vi "HELP.vi"(0 "System no.":i32=1 min=1 max=4 step=1, 5 "error in":errorcluster) -> (14 "Help string":string, 19 "error out":errorcluster)   [LabVIEW 2026]
doc: "Returns help string.\n\nF-206, M-8X0: Only for GCS syntax version = GCS 1.0 (Check with CSV?.vi. If CSV?.vi is not supported, syntax version is GCS 1.0). For GCS 2.0 use HLP?.vi instead."
uses:
  GeneralCommands/Controller names.ctl
  Communication/Syntax.ctl
  Communication/Global1.vi
  GeneralCommands/Global2 (Array).vi
panel:
  # "Get  help (new command: HLP?)."
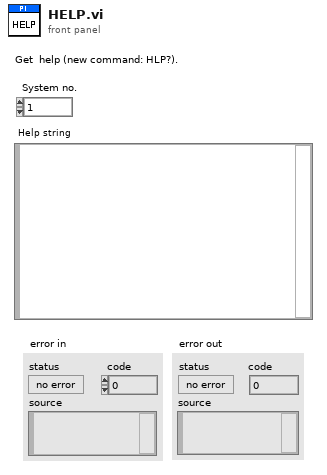
[diagram p1: front panel]
types:
  T1 = typedef "Syntax.ctl" = enum16{"GCS 1.0", "GCS 2.0", "GCS 3.0"}
  T2 = typedef "Controller names.ctl" = enum16{"None", "Analog", "C-702", "C-413", "C-414", "C-843", "C-843.PM", "C-844", "C-848", "C-865", "C-866", "C-867", "C-877", "C-880", "C-884", "C-885", "C-886", "C-887", "C-891", "E-135", "E-516", "E-517", "E-518", "E-709", "E-710", "E-712", "E-725", "E-727", "E-753", "E-754", "E-755", "E-761", "E-816", "E-861", "E-870", "E-871", "E-872", "E-873", "E-874", "F-206", "HydraPollux", "M-840", "M-850", "M-8X0", "Mercury", "Mercury_GCS", "PI_GCS2"}
  T3 = cluster{"Conn. axes":string[], "Controller name":T2}[]
  T4 = cluster{"Conn. axes":string[], "Controller name":T2}
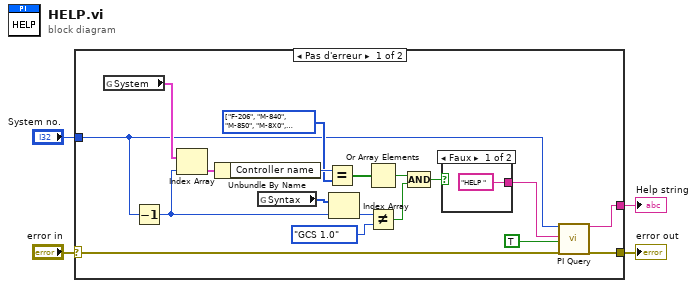
[diagram p0: block diagram]
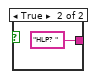
[diagram p2: hidden frame]
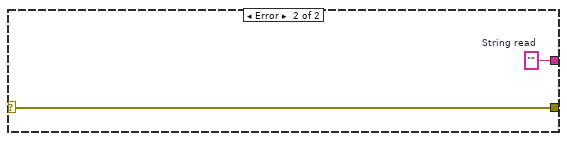
[diagram p3: hidden frame]
diagram:
  n1 = case shown="Pas d'erreur" "error in" {
    selector: "error in" -> [w8 w26]
    tunnel: [w6 w25] -> w4
    tunnel: [w7 w26] -> w3
    tunnel: "System no." -> [w10 _]
    frame No Error {
      w15 = T2[] [enum."F-206", enum."M-840", enum."M-850", enum."M-8X0", enum."C-887"] items=["None", "Analog", "C-702", "C-413", "C-414", "C-843", "C-843.PM", "C-844", "C-848", "C-865", "C-866", "C-867", "C-877", "C-880", "C-884", "C-885", "C-886", "C-887", "C-891", "E-135", "E-516", "E-517", "E-518", "E-709", "E-710", "E-712", "E-725", "E-727", "E-753", "E-754", "E-755", "E-761", "E-816", "E-861", "E-870", "E-871", "E-872", "E-873", "E-874", "F-206", "HydraPollux", "M-840", "M-850", "M-8X0", "Mercury", "Mercury_GCS", "PI_GCS2"]
      n2 = global read "Global2 (Array).vi" "System"() -> (w19:T3)
      n3 = Decrement(x=w10) -> (x-1=w18:i32)
      n4 = Index Array(array=w19, index=w18) -> (element=w17:T4)
      n5 = Unbundle By Name(w17) -> ("Controller name"=w16:T2)
      n6 = global read "Global1.vi" "Syntax"() -> (w21:T1[])
      n7 = Equal?(x=w16, y=w15) -> (x = y?=w14:bool[])
      n8 = Index Array(array=w21, index=w18) -> (element=w20:T1)
      n9 = Or Array Elements(Boolean array=w14) -> (logical OR=w13:bool)
      n10 = Not Equal?(x=w20, y=Syntax."GCS 1.0") -> (x != y?=w12:bool)
      n11 = Compound Arithmetic op=AND(w13, w12) -> (w11:bool)
      n12 = case shown="Faux" w11 {
        tunnel: ["HELP " "HLP? "] -> w9
        frame False {
        }
        frame True {
        }
      }
      n13 = call "PI Query.vi"("System no."=w10, "String to send"=w9, "Attach termination char.?"=TRUE ("Attach Linefeed?"), "error in"=w8) -> ("String read"=w6:string, "error out"=w7:errorcluster)  [unwired: 3 in, 11 out]
    }
    frame Error {
      w25 = ""  # String read
    }
  }
  "Help string" <- w4
  "error out" <- w3
